vi "PDA_Spectral_Acquisition.vi"(1 "Shutter":bool=TRUE, 2 "Number of Regions":u32=1, 3 "Number of Cycles":u32=1 min=1 max=30, 4 "Acquisition Parameters":T2={"Exposure (ms)"=100, "Interval (ms)"=10, "Flush Count"=1, "Trigger"=0} {"Trigger" items=["Disable", "Acquistion", "Cycle"]}) -> (5 "Display":sgl[][](graph), 6 "Acq Busy":bool, 7 "Read count":u32=1 min=1 max=30)   [LabVIEW 2021]
doc: "This VI demonstrates acquisition and image display of CCD data\nutilizing the ISA CCD driver.\n\nNote: Specific help is available for each individual control, display and indicator."
uses:
  IGA_comm.llb/Controller Version Number.vi
panel:
  out "Current Operation":T1(ring)
  in  "Gain":bool
  out "error out":errorcluster
  in  "error in":errorcluster
  in  "StartIng Mode":T1(ring)
  in  "Number of Region copy":u32=4
  in  "stop":bool
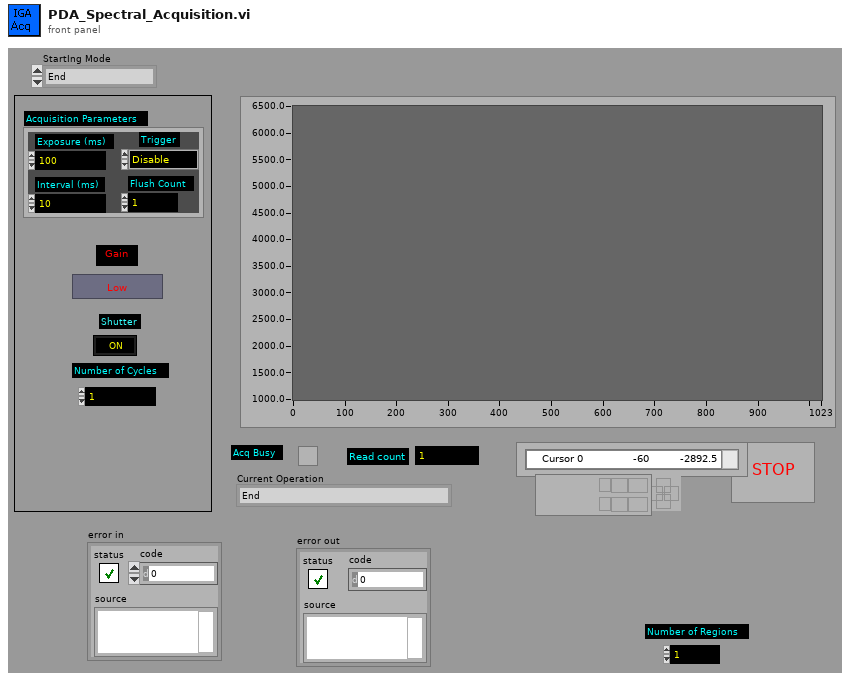
[diagram p1: front panel]
types:
  T1 = enum16{"End", "Init", "Reset", "SetAcqParameter", "SetArea", "Start Acquisition", "Busy Status Poll", "Read", "Stop"}
  T2 = cluster{"Exposure (ms)":u32, "Interval (ms)":u32, "Flush Count":i32, "Trigger":u16}
  T3 = cluster{"Comm Interface":u16, "BUS":i16, "Address":i16, "Com Port":i32}
  T4 = cluster{"X Origin":u32, "Y Origin":u32, "X Size":u32, "Y Size":u32, "X Bin":u32, "Y Bin":u32}[]
  T5 = cluster{"Exposure (ms)":bool, "Interval (ms)":bool, "Flush Count":bool, "Trigger":bool}
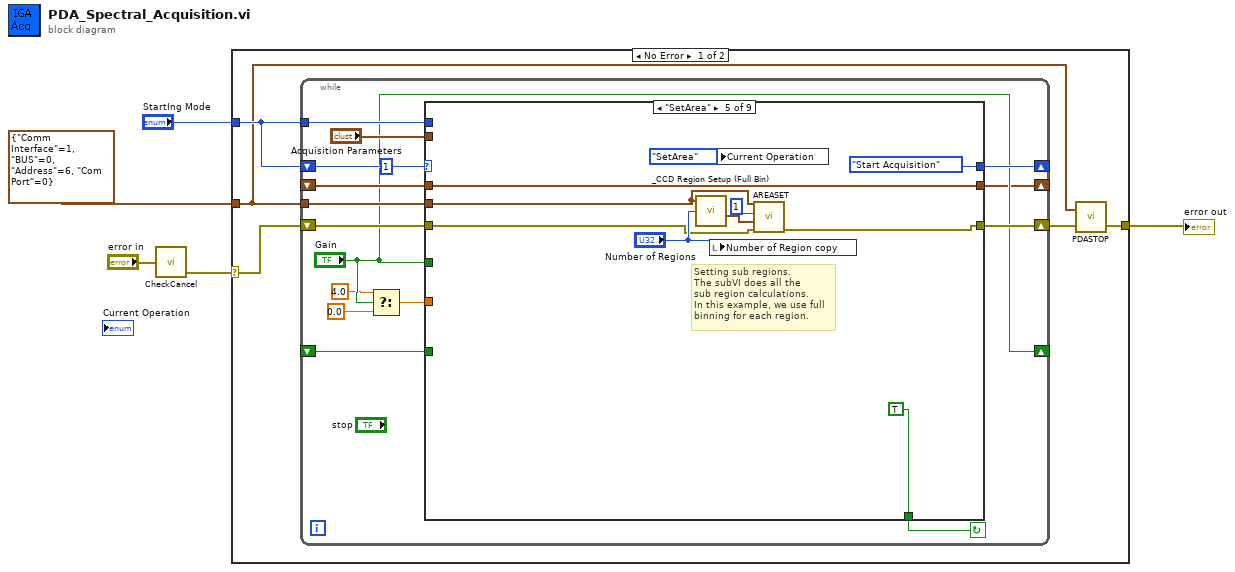
[diagram p0: block diagram]
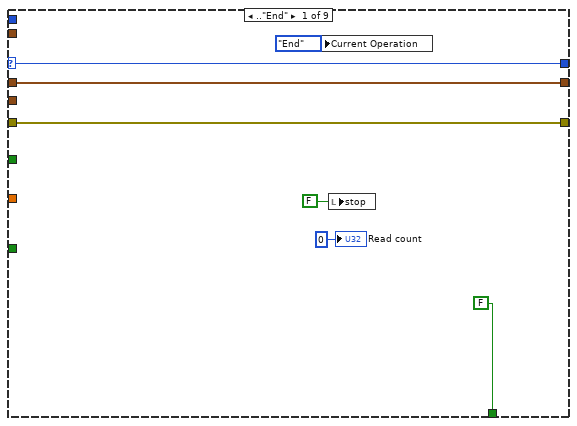
[diagram p2: hidden frame]
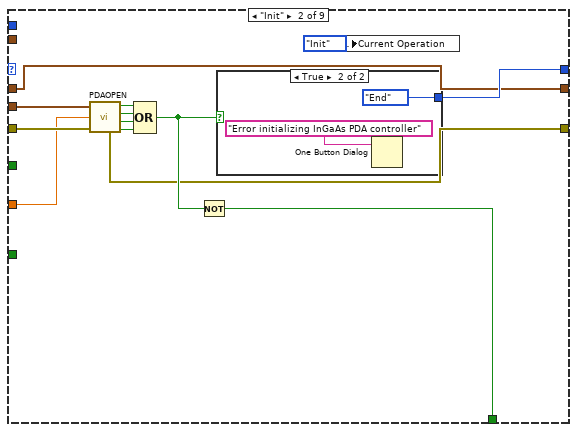
[diagram p3: hidden frame]
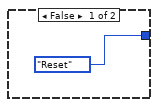
[diagram p4: hidden frame]
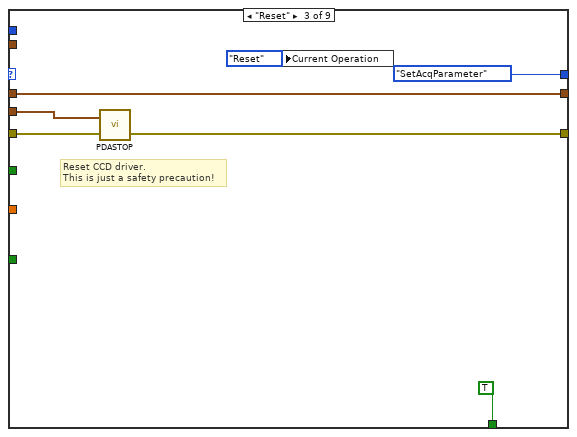
[diagram p5: hidden frame]
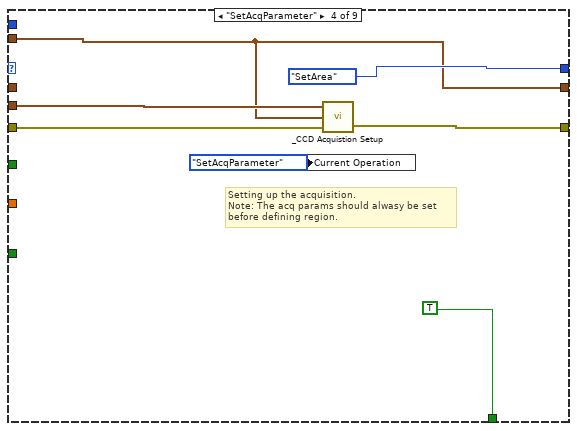
[diagram p6: hidden frame]
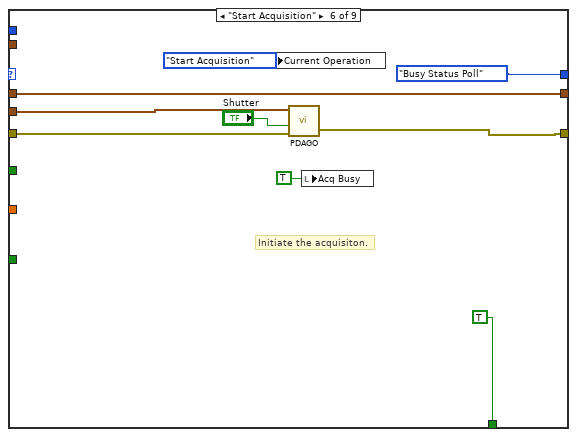
[diagram p7: hidden frame]
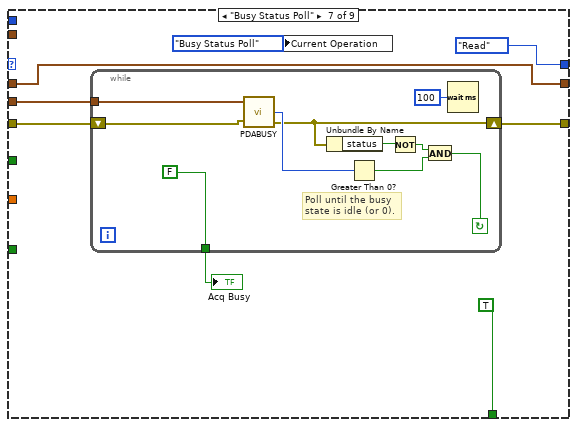
[diagram p8: hidden frame]
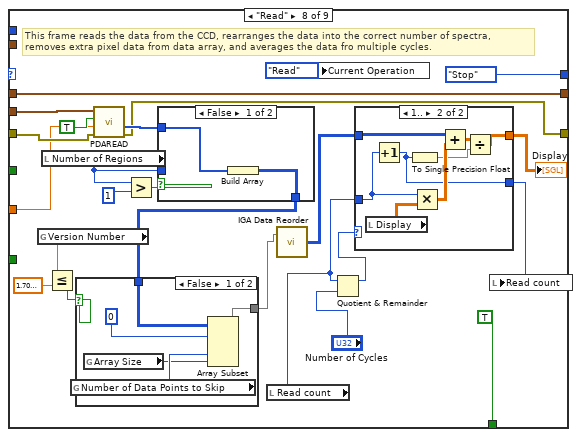
[diagram p9: hidden frame]
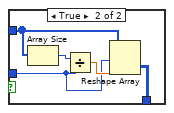
[diagram p11: hidden frame]
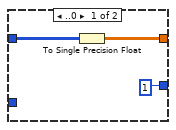
[diagram p12: hidden frame]
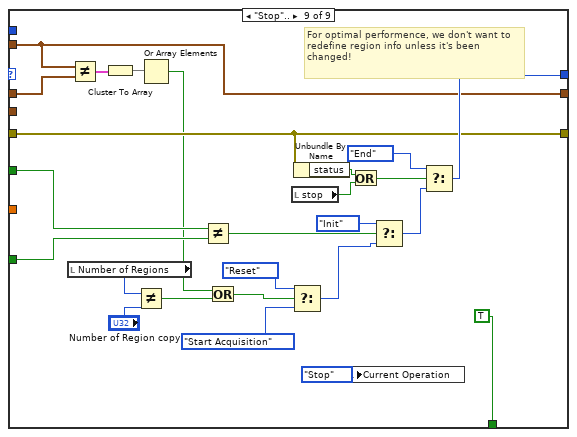
[diagram p13: hidden frame]
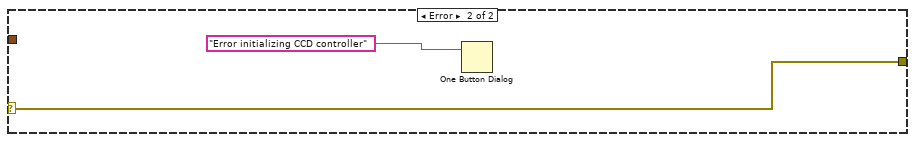
[diagram p14: hidden frame]
diagram:
  n1 = call "CheckCancel.vi"("error in (no error)"="error in") -> ("error out"=w3:errorcluster)  [unwired: 1 in, 1 out]
  n2 = case shown="No Error" w3 {
    selector: w3 -> [w10 w173]
    tunnel: T3 {"Comm Interface"=1, "BUS"=0, "Address"=6, "Com Port"=0} ("Comm Params") -> [w6 _]
    tunnel: "StartIng Mode" -> [w8 _]
    tunnel: [w7 w173] -> w1
    frame No Error {
      (unwired) 1
      n3 = while {
        shift-left: w10 -> [w23]
        shift-right: [w24] -> w9
        tunnel: w6 -> [w22]
        shift-right: [w11] -> _
        shift-left: _ -> [w21]
        tunnel: w8 -> [w20]
        shift-right: ["Gain"] -> _
        shift-left: _ -> [w19]
        shift-right: [w18] -> _
        shift-left: w8 -> [w17]
        stop <- w25 continue-if-true
        n4 = Select(t=4.0, s="Gain", f=0.0) -> (s? t:f=w14:dbl)
        n5 = case shown="\"SetArea\"" w17 {
          selector: w17 -> [w30 _ _ _ _ _ _ _ _]
          tunnel: [FALSE w38 TRUE TRUE TRUE TRUE TRUE TRUE TRUE] -> w25
          tunnel: [w30 w36 T1."SetAcqParameter" ("StartIng Mode") T1."SetArea" ("StartIng Mode") T1."Start Acquisition" ("StartIng Mode") T1."Busy Status Poll" ("StartIng Mode") T1."Read" ("StartIng Mode") T1."Stop" ("StartIng Mode") w169] -> w18
          tunnel: w23 -> [w29 w41 w53 w60 w66 w79 w88 w105 w167]
          tunnel: [w29 w37 w52 w59 w65 w78 w86 w104 w167] -> w24
          tunnel: "Gain" -> [_ _ _ _ _ _ _ _ w163]
          tunnel: w22 -> [_ w40 w51 w61 w67 w77 w87 w106 _]
          tunnel: w21 -> [w27 w34 w50 _ w64 w74 w83 w101 w152]
          tunnel: w20 -> [_ _ _ _ _ _ _ _ _]
          tunnel: w19 -> [_ _ _ _ _ _ _ _ w162]
          tunnel: "Acquisition Parameters" -> [_ _ _ w57 _ _ _ _ w149]
          tunnel: w14 -> [_ w35 _ _ _ _ _ w102 _]
          tunnel: [w27 w34 w50 w57 w64 w74 w83 w101 w149] -> w11
          frame .."End" {
            n6 = local write "Current Operation"(T1."End" ("Current Operation")) -> ()
            n7 = local write "stop"(FALSE ("stop")) -> ()
            "Read count" <- u32 0 ("Read count")
          }
          frame "Init" {
            n8 = call "PDAOPEN.VI"("error in"=w41, "CCD ADC and Gain"=w35, "Comm Params"=w40) -> ("State Error"=w42:bool, "error out"=w37:errorcluster, "Table Error"=w43:bool, "Init Error"=w44:bool, "Boot Error"=w45:bool)  [unwired: 1 out]
            n9 = Compound Arithmetic op=OR(w45, w44, w43, w42) -> (w39:bool)
            n10 = Not(x=w39) -> (.not. x?=w38:bool)
            n11 = case shown="True" w39 {
              tunnel: [T1."Reset" ("StartIng Mode") T1."End" ("StartIng Mode")] -> w36
              frame False {
              }
              frame True {
                n12 = One Button Dialog(message="Error initializing InGaAs PDA controller") -> ()  [unwired: 1 in, 1 out]
              }
            }
            n13 = local write "Current Operation"(T1."Init" ("Current Operation")) -> ()
          }
          frame "Reset" {
            # "Reset CCD driver.\nThis is just a safety precaution!"
            n14 = call "PDASTOP.VI"("error in"=w53, "Comm Params"=w51) -> ("error out"=w52:errorcluster)  [unwired: 1 out]
            n15 = local write "Current Operation"(T1."Reset" ("Current Operation")) -> ()
          }
          frame "SetAcqParameter" {
            # "Setting up the acquisition.\nNote: The acq params should alwasy be set\nbefore defining region."
            n16 = local write "Current Operation"(T1."SetAcqParameter" ("Current Operation")) -> ()
            n17 = call "_CCD Acquistion Setup.vi"("error in"=w60, "Acquisition Param"=w57, "Comm Params"=w61) -> ("error out"=w59:errorcluster)  [unwired: 1 out]
          }
          frame "SetArea" {
            # "Setting sub regions.\nThe subVI does all the\nsub region calculations.\nIn this example, we use full\nbinning for each region."
            n18 = call "_CCD Region Setup (Full Bin).vi"("Comm Params"=w67, "Number of Regions"="Number of Regions") -> ("Region Info Array"=w70:T4)  [unwired: 1 in, 3 out]
            n19 = local write "Number of Region copy"("Number of Regions") -> ()
            n20 = local write "Current Operation"(T1."SetArea" ("Current Operation")) -> ()
            n21 = call "AREASET.VI"("error in"=w66, "Region Info Array"=w70, "Acquisition Format"=1, "Comm Params"=w67) -> ("error out"=w65:errorcluster)  [unwired: 3 in, 1 out]
          }
          frame "Start Acquisition" {
            # "Initiate the acquisiton."
            n22 = local write "Current Operation"(T1."Start Acquisition" ("Current Operation")) -> ()
            n23 = call "PDAGO.VI"("error in"=w79, "Shutter"="Shutter", "Comm Params"=w77) -> ("error out"=w78:errorcluster)  [unwired: 1 in, 1 out]
            n24 = local write "Acq Busy"(TRUE ("Acq Busy")) -> ()
          }
          frame "Busy Status Poll" {
            n25 = while {
              shift-right: [w95] -> w86
              shift-left: w88 -> [w97]
              tunnel: w87 -> [w96]
              tunnel: [FALSE ("Acq Busy")] -> w84
              stop <- w91 continue-if-true
              # "Poll until the busy\nstate is idle (or 0)."
              n26 = call "PDABUSY.VI"("Comm Params"=w96, "error in"=w97) -> ("CCD Status"=w99:u16, "error out"=w95:errorcluster)  [unwired: 1 out]
              n27 = Unbundle By Name(w95) -> ("status"=w94:bool)
              n28 = Greater Than 0?(x=w99) -> (x > 0?=w92:bool)
              n29 = Not(x=w94) -> (.not. x?=w93:bool)
              n30 = And(x=w93, y=w92) -> (x .and. y?=w91:bool)
              n31 = Wait (ms)(milliseconds to wait=u32 100) -> ()  [unwired: 1 out]
            }
            "Acq Busy" <- w84
            n32 = local write "Current Operation"(T1."Busy Status Poll" ("Current Operation")) -> ()
          }
          frame "Read" {
            # "This frame reads the data from the CCD, rearranges the data into the correct number of spectra, \nremoves extra pixel data from data array, and averages the data fro multiple cycles."
            n33 = global read "Controller Version Number.vi" "Version Number"() -> (w112:sgl)
            n34 = local read "Number of Regions"() -> (w117:u32)
            n35 = Less Or Equal?(x=w112, y=sgl 1.7) -> (x <= y?=w110:bool)
            n36 = call "PDAREAD.VI"("Comm Params"=w106, "Reset Image?"=TRUE, "CCD ADC and Gain"=w102, "error in"=w105) -> ("Data"=w116:u16[], "error out"=w104:errorcluster)  [unwired: 3 out]
            n37 = Greater?(x=w117, y=u32 1) -> (0:w115:bool)
            n38 = case shown="False" w115 {
              tunnel: w116 -> [w130 w135]
              tunnel: [w131 w136] -> w109
              tunnel: w117 -> [_ w132]
              frame False {
                n39 = Build Array(w130) -> (w131:u16[][])
              }
              frame True {
                n40 = Array Size(array=w135) -> (size(s)=w134:i32)
                n41 = Divide(x=w134, y=w132) -> (x/y=w133:dbl)
                n42 = Reshape Array(w135, w132, w133) -> (w136:u16[][])
              }
            }
            n43 = case shown="False" w110 {
              tunnel: w109 -> [w128 w129]
              tunnel: [w127 w129] -> w108
              frame False {
                n44 = global read "Controller Version Number.vi" "Number of Data Points to Skip"() -> (w126:i8)
                n45 = global read "Controller Version Number.vi" "Array Size"() -> (w125:i32)
                n46 = Array Subset(array=w128, index (row)=0 ("Array Index"), index (col)=w126, length (col)=w125) -> (w127:u16[][])  [unwired: 1 in]
              }
              frame True {
              }
            }
            n47 = local read "Read count"() -> (w120:u32)
            n48 = call "IGA Data Reorder.VI"("Input Array"=w108) -> ("Output Array"=w107:i32[][])  [unwired: 2 in]
            n49 = local write "Current Operation"(T1."Read" ("Current Operation")) -> ()
            n50 = Quotient & Remainder(x=w120, y="Number of Cycles") -> (x-y*floor(x/y)=w122:u32)  [unwired: 1 out]
            n51 = case shown="1.." w122 {
              tunnel: w107 -> [w139 w146]
              tunnel: [w138 w142] -> w121
              tunnel: w120 -> [_ w141]
              tunnel: [u32 1 ("Read count") w140] -> w118
              frame ..0 {
                n52 = To Single Precision Float(number=w139) -> (single precision float=w138:sgl[][])
              }
              frame 1.. {
                n53 = local read "Display"() -> (w147:sgl[][])
                n54 = Increment(x=w141) -> (x+1=w140:u32)
                n55 = To Single Precision Float(number=w140) -> (single precision float=w143:sgl)
                n56 = Multiply(x=w141, y=w147) -> (x*y=w145:sgl[][])
                n57 = Add(x=w146, y=w145) -> (x+y=w144:sgl[][])
                n58 = Divide(x=w144, y=w143) -> (x/y=w142:sgl[][])
              }
            }
            "Display" <- w121
            n59 = local write "Read count"(w118) -> ()
          }
          frame "Stop".. {
            # "For optimal performence, we don't want to redefine region info unless it's been changed!"
            n60 = local read "Number of Regions"() -> (w171:u32)
            n61 = Not Equal?(x=w149, y=w152) -> (x != y?=w154:T5)
            n62 = Cluster To Array(cluster=w154) -> (array=w153:bool[])
            n63 = Not Equal?(x=w171, y="Number of Region copy") -> (x != y?=w151:bool)
            n64 = Or Array Elements(Boolean array=w153) -> (logical OR=w155:bool)
            n65 = Not Equal?(x=w163, y=w162) -> (x != y?=w161:bool)
            n66 = Or(x=w155, y=w151) -> (x .or. y?=w150:bool)
            n67 = local read "stop"() -> (w165:bool)
            n68 = Select(t=T1."Reset" ("StartIng Mode"), s=w150, f=T1."Start Acquisition") -> (s? t:f=w157:T1)
            n69 = Unbundle By Name(w167) -> ("status"=w166:bool)
            n70 = local write "Current Operation"(T1."Stop" ("Current Operation")) -> ()
            n71 = Or(x=w166, y=w165) -> (x .or. y?=w164:bool)
            n72 = Select(t=T1."Init" ("StartIng Mode"), s=w161, f=w157) -> (s? t:f=w156:T1)
            n73 = Select(t=T1."End" ("StartIng Mode"), s=w164, f=w156) -> (s? t:f=w169:T1)
          }
        }
      }
      n74 = call "PDASTOP.VI"("error in"=w9, "Comm Params"=w6) -> ("error out"=w7:errorcluster)  [unwired: 1 out]
    }
    frame Error {
      n75 = One Button Dialog(message="Error initializing CCD controller") -> ()  [unwired: 1 in, 1 out]
    }
  }
  "error out" <- w1
